vi "Database Logging.vi"() -> ()   [LabVIEW 2012]
doc: "This example inserts data into a table named logging in the LabVIEW.mdb database. The data is generated and inserted into the database once per second until you press the Stop button. You can use either of the Playback examples to read the data back into LabVIEW.\n\nThe diagram is easy to use because you only need three Database Tools subVIs - DB Tools Open Connection, DB Tools Insert Data, and DB Tools Close Connection. To insert the data, you do not need to use SQL commands or worry about defining or converting data types. You bundle all the data into a cluster and wire that cluster to the DB Tools Insert Data VI."
uses:
  Connection.llb/DB Tools Open Connec (Path).vi
  NI_Database_API_64.lvlib
panel:
  out "Number of Records":i32
  in  "stop":bool
  out "min temperature value":dbl format="%.2f"
  out "max temperature value":dbl format="%.2f"
  out "min pressure value":dbl format="%.2f"
  out "max pressure value":dbl format="%.2f"
  out "Core Temperature":dbl[](graph)
  out "Core Pressure":dbl[](graph)
  out "Core Measuments":dbl[][](graph)
  # "INSTRUCTIONS:\n\nRun the VI to insert data \ninto a table called logging \nin the example database - \nLabVIEW.mdb.  \nYou can then use the \nPlayback VIs to read the \ndata back into LabVIEW."
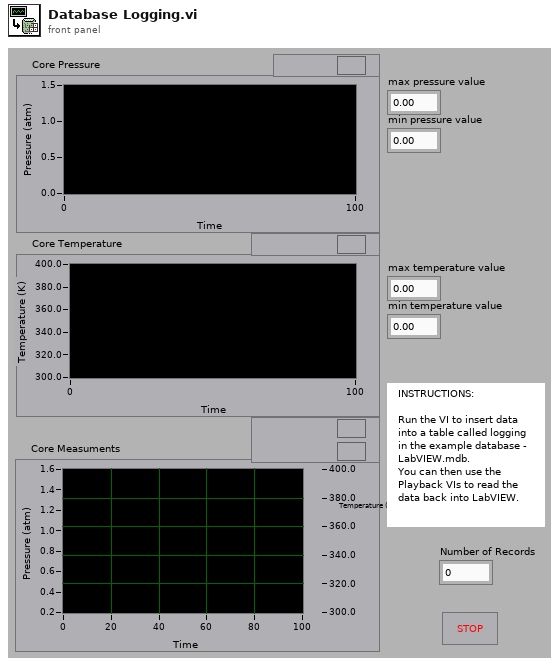
[diagram p1: front panel]
types:
  T1 = typedef "NI_Database_API_64.lvlib/Conn ObjectReference.ctl" = refnum<k1>
  T2 = cluster{i32, "core pressure":dbl[], dbl, dbl, "core temperature":dbl[], dbl, dbl}
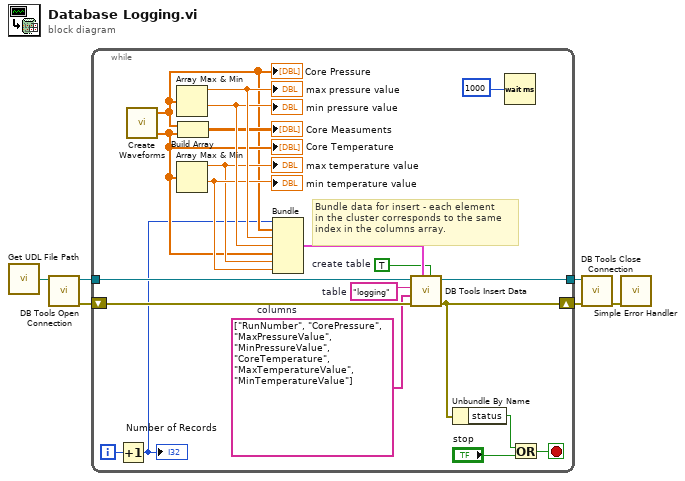
[diagram p0: block diagram]
diagram:
  n1 = call "Get UDL File Path.vi"() -> ("UDL file path"=w1:path)  [unwired: 1 in]
  n2 = call-poly "DB Tools Open Connection.vi"("connection information"=w1) -> ("error out"=w5:errorcluster, "connection reference"=w6:T1)  [unwired: 7 in]
  n3 = while {
    tunnel: w6 -> [w20]
    tunnel: [w21] -> w4
    shift-right: [w15] -> w3
    shift-left: w5 -> [w19]
    i -> [w22]
    stop <- w12 stop-if-true
    w7 = string[] ["RunNumber", "CorePressure", "MaxPressureValue", "MinPressureValue", "CoreTemperature", "MaxTemperatureValue", "MinTemperatureValue"]  # columns
    w18 = "logging"  # table
    w16 = TRUE  # create table
    # "Bundle data for insert - each element \nin the cluster corresponds to the same \nindex in the columns array."
    n4 = Increment(x=w22) -> (x+1=w8:i32)
    "Number of Records" <- w8
    n5 = call "Create Waveforms.vi"() -> ("core pressure"=w9:dbl[], "core temperature"=w10:dbl[])  [unwired: 3 in]
    "Core Pressure" <- w9
    "Core Temperature" <- w10
    n6 = Array Max & Min(array=w9) -> (max value=w27:dbl, min value=w26:dbl)  [unwired: 2 out]
    "max pressure value" <- w27
    "min pressure value" <- w26
    n7 = Array Max & Min(array=w10) -> (max value=w23:dbl, min value=w25:dbl)  [unwired: 2 out]
    "max temperature value" <- w23
    "min temperature value" <- w25
    n8 = Build Array(w9, w10) -> (→"Core Measuments":dbl[][])
    n9 = Bundle(w8, "core pressure"=w9, w27, w26, "core temperature"=w10, w23, w25) -> (w17:T2)  [unwired: 1 in]
    n10 = call "DB Tools Insert Data.vi"("create table? (F)"=w16, "data"=w17, "error in (no error)"=w19, "columns"=w7, "table"=w18, "connection reference"=w20) -> ("error out"=w15:errorcluster, "connection reference out"=w21:T1)  [unwired: 4 in]
    n11 = Unbundle By Name(w15) -> ("status"=w14:bool)
    n12 = Wait (ms)(milliseconds to wait=u32 1000) -> ()  [unwired: 1 out]
    n13 = Or(x=w14, y="stop") -> (x .or. y?=w12:bool)
  }
  n14 = call "DB Tools Close Connection.vi"("error in (no error)"=w3, "connection reference"=w4) -> ("error out"=w2:errorcluster)  [unwired: 5 in]
  n15 = call <vilib>:"Simple Error Handler.vi"("error in (no error)"=w2) -> ()  [unwired: 4 in, 5 out]
